vi "harp_write_R_MEMORY.vi"(0 "port":refnum<visa-resource-name>, 11 "error in (no error)":errorcluster, 13 "reset mode":u16(ring)=1 items=["B_RST_DEF"=1, "B_RST_EE"=2, "B_RST_SAVE"=4, "B_NAME_TO_DEFAULT"=8]) -> (4 "port out":refnum<visa-resource-name>, 15 "error out":errorcluster)   [LabVIEW 2010]
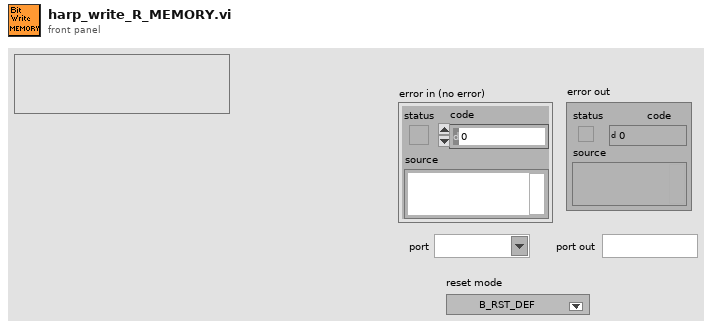
[diagram p1: front panel]
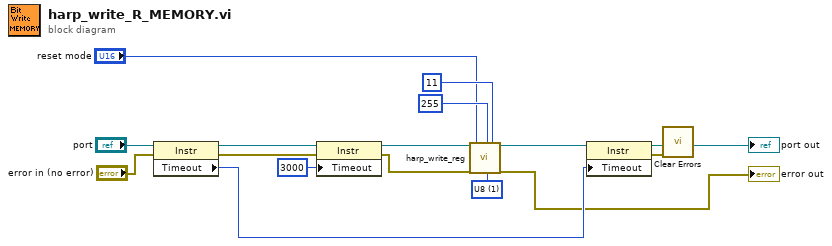
[diagram p0: block diagram]
diagram:
  w15 = u8 1 items=["U8"=1, "U16"=2, "U32"=4, "U64"=8, "I8"=129, "I16"=130, "I32"=132, "I64"=136, "FLOAT"=68, "BOOL"=17] ("type")
  n1 = property class="Instr"(reference="port", error in="error in (no error)") -> (reference out=w11:refnum<visa-resource-name>, error out=w10:errorcluster, "Timeout"=w5:u32)
  n2 = property class="Instr"(reference=w11, error in=w10, "Timeout"=u32 3000 ("General Settings:Timeout Value")) -> (reference out=w8:refnum<visa-resource-name>, error out=w7:errorcluster)
  n3 = call "harp_write_reg.vi"(0:"port"=w8, "error in (no error)"=w7, "8 bits"="reset mode", 10:"port"=u8 255 ("port"), "type"=w15, "reg. address"=u8 11) -> ("port out"=w6:refnum<visa-resource-name>, "error out"=→"error out":errorcluster)  [unwired: 11 in, 1 out]
  n4 = property class="Instr"(reference=w6, "Timeout"=w5) -> (reference out=→"port out":refnum<visa-resource-name>, error out=w1:errorcluster)  [unwired: 1 in]
  n5 = call <vilib>:"Clear Errors.vi"("error in (no error)"=w1) -> ()  [unwired: 6 in, 1 out]
